vi "To String.vi"(8 "error in (no error)":errorcluster, 11 "Path Array in":refnum<class "Path Array.lvclass">) -> (0 "error out":errorcluster, 2 "String":string)   [LabVIEW 2020, in "Data.lvlib" / "Path Array.lvclass"]
doc: "Convert 'Generic Data in' to a string."
uses:
  Path Array.lvclass
  Path Array.lvclass/Path Array.ctl
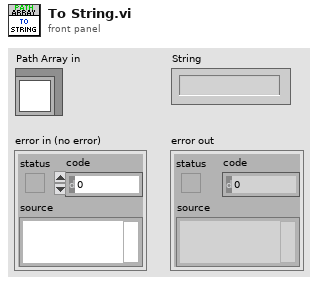
[diagram p1: front panel]
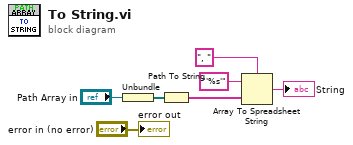
[diagram p0: block diagram]
diagram:
  n1 = Unbundle("Path Array in") -> (w5:path[])
  n2 = Path To String(path=w5) -> (string=w1:string[])
  n3 = Array To Spreadsheet String(delimiter (Tab)=", ", array=w1, 3:"'%s'" ("format string")) -> (spreadsheet string=→"String":string)
  "error out" <- "error in (no error)"
